vi "Set Slew.vi"(8 "error in (no error)":errorcluster, 9 "Slew (V/s)":dbl, 10 "Output Channel":T1, 11 "VISA resource name":refnum<visa-resource-name>) -> (0 "error out":errorcluster, 2 "Output Channel":T1, 3 "VISA Refnum out":refnum<visa-resource-name>)   [LabVIEW 2019, in "RP100.lvlib"]
uses:
  RP100.lvlib
  Inst.RP100/Typedefs/Channel--Num.ctl
  Inst.RP100/Inst.RP100.lvclass
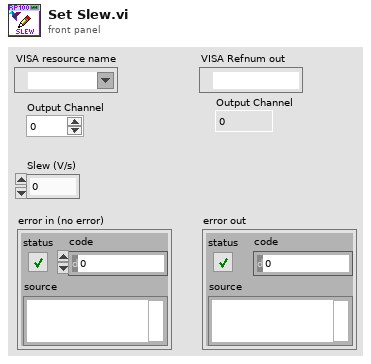
[diagram p1: front panel]
types:
  T1 = typedef "Inst.RP100.lvlib/Inst.RP100.lvclass/Channel--Num.ctl" = i32
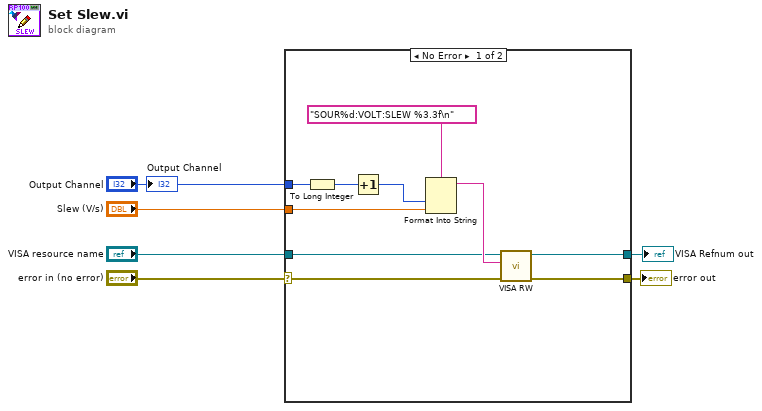
[diagram p0: block diagram]
diagram:
  n1 = case shown="No Error" "error in (no error)" {
    selector: "error in (no error)" -> [w11 w18]
    tunnel: [w9 w17] -> w6
    tunnel: [w10 w18] -> w5
    tunnel: "Slew (V/s)" -> [w16 _]
    tunnel: "VISA resource name" -> [w12 w17]
    tunnel: "Output Channel" -> [w15 _]
    frame No Error {
      n2 = To Long Integer(number=w15) -> (32bit integer=w8:T1)
      n3 = Increment(x=w8) -> (x+1=w7:T1)
      n4 = Format Into String(format string="SOUR%d:VOLT:SLEW %3.3f\n", w7, w16) -> (resulting string=w13:string)  [unwired: 2 in, 1 out]
      n5 = call "VISA RW.vi"("error in (no error)"=w11, "Write"=w13, "VISA Refnum in"=w12) -> ("error out"=w10:errorcluster, "VISA Refnum out"=w9:refnum<visa-resource-name>)  [unwired: 6 in, 1 out]
    }
    frame Error {
    }
  }
  "VISA Refnum out" <- w6
  "error out" <- w5
  "Output Channel" <- "Output Channel"
